vi "File List Window 2.vi"(8 "error in":errorcluster, 9 "File Type":T1=enum."Build Spec (vipb)", 11 "Path":path=path "C:/Users/patrick/AppData/Local/LevyLab/build-support/instruments-vipb--lockin.txt") -> (0 "error out":errorcluster, 1 "File Type out":T1=enum."Build Spec (vipb)", 2 "files out":path[](array[path]), 3 "Path out":path=path "C:/Users/patrick/AppData/Local/LevyLab/build-support/instruments-vipb--lockin.txt")   [LabVIEW 2019, in "Build.lvlib"]
uses:
  Typedefs/Build Type--enum.ctl
  <vilib>/Utility/sysdir.llb/System Directory Type.ctl
  <vilib>/Utility/file.llb/Write Delimited Spreadsheet (string).vi
  <vilib>/Utility/file.llb/Read Delimited Spreadsheet (string).vi
  Build.lvlib
panel:
  in  "Cancel":bool
  in  "OK":bool
  in  "Paths":path[](array[path])
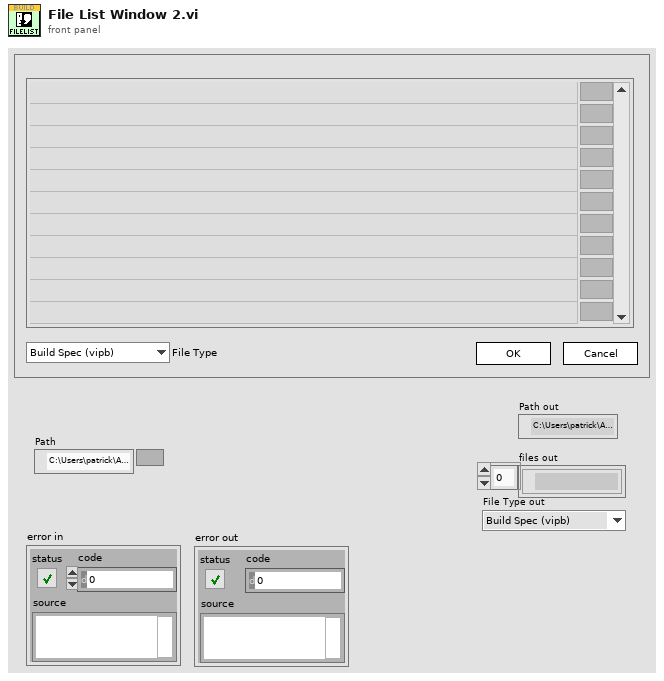
[diagram p1: front panel]
types:
  T1 = typedef "Build.lvlib/Build Type--enum.ctl" = enum16{"LV Project (lvproj)", "Build Spec (vipb)", "Package (vip)"}
  T2 = enum32{"Invalid", "Standard", "Closed", "Hidden", "Minimized", "Maximized"}
  T3 = enum32{"invalid app kind", "Development System", "Run Time System", "Student Edition", "Embedded LabVIEW", "Evaluation", "Custom"}
  T4 = cluster{"Core":cluster{"Current VI Reference":refnum<vi>, "Close Panel on Exit?":bool}, "Path":path, "files":path[], "File Type":T1}
  T5 = typedef "System Directory Type.ctl" = i32
  T6 = cluster{"Current VI Reference":refnum<vi>, "Close Panel on Exit?":bool}
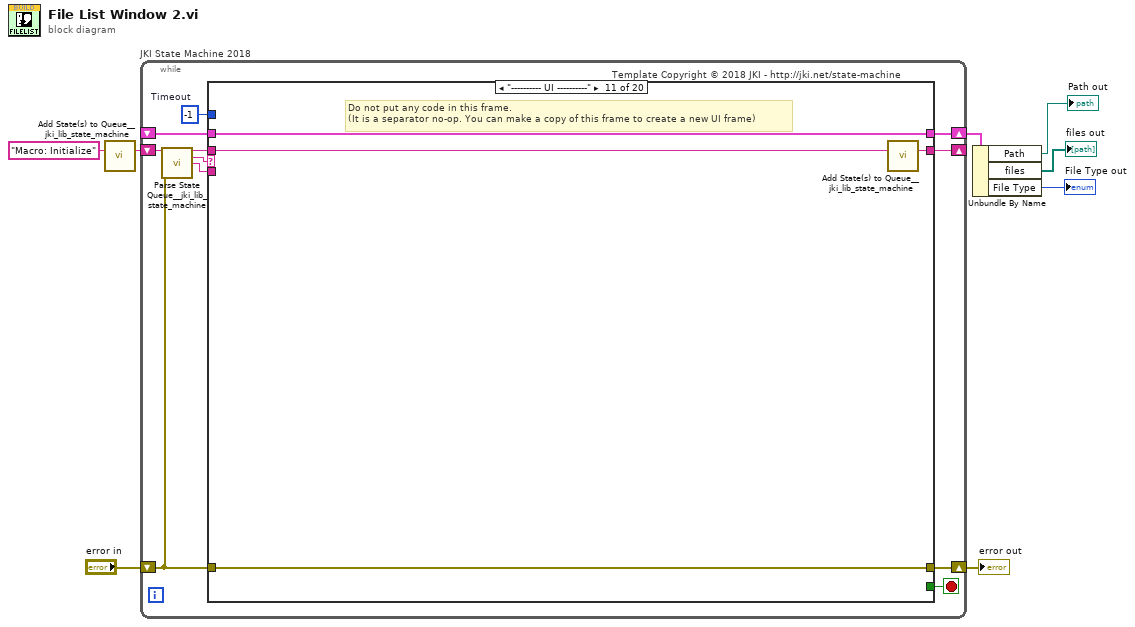
[diagram p0: block diagram]
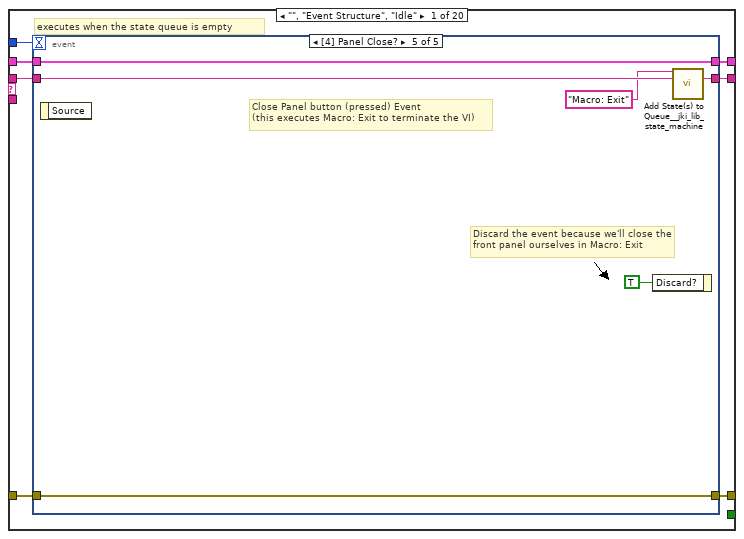
[diagram p2: hidden frame]
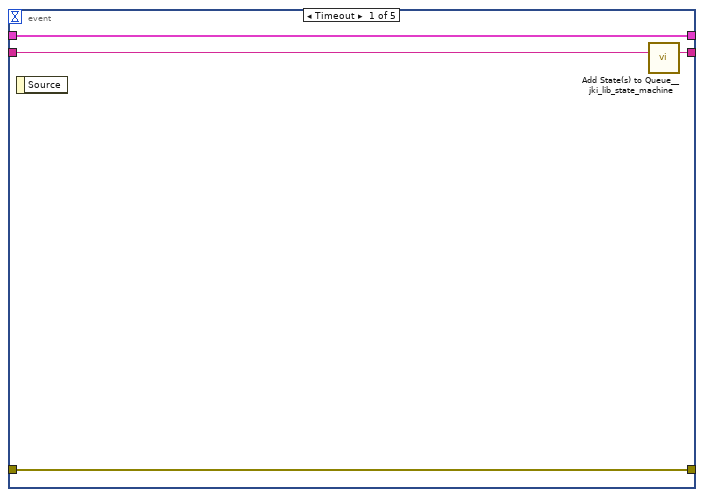
[diagram p3: hidden frame]
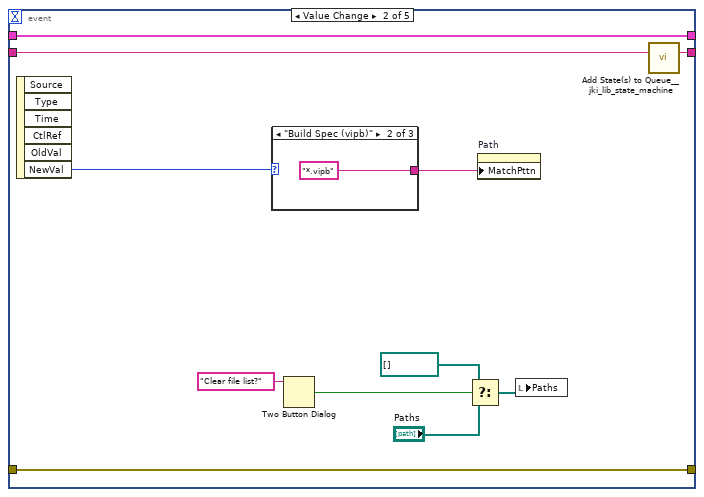
[diagram p4: hidden frame]
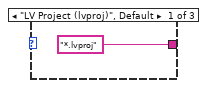
[diagram p5: hidden frame]
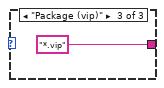
[diagram p6: hidden frame]
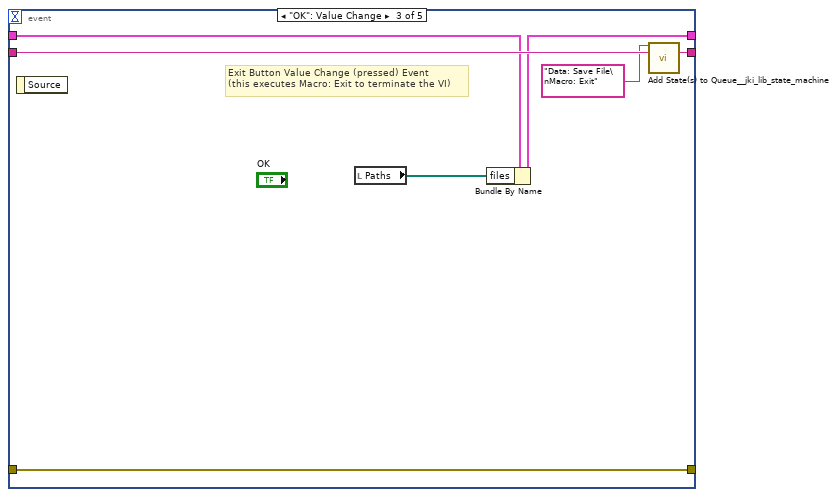
[diagram p7: hidden frame]
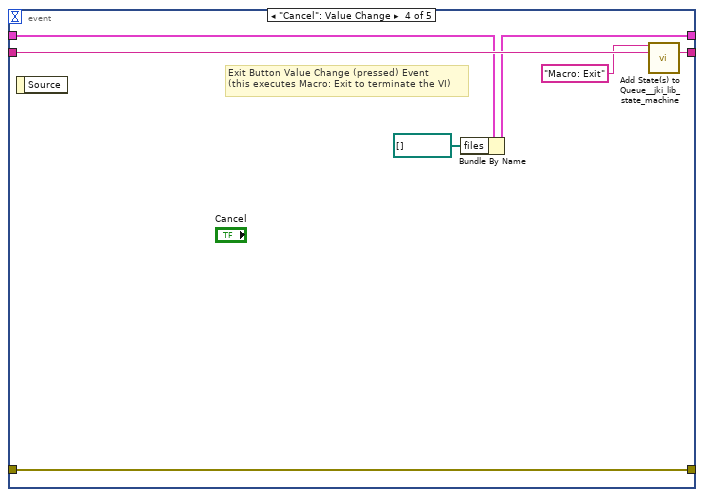
[diagram p8: hidden frame]
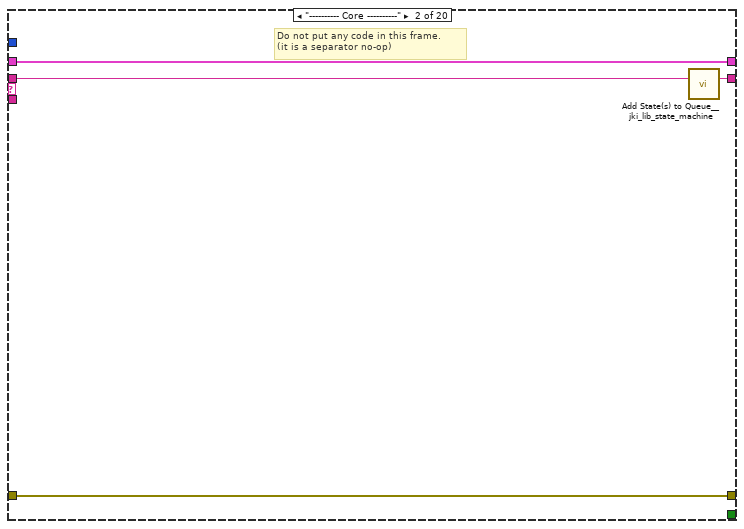
[diagram p9: hidden frame]
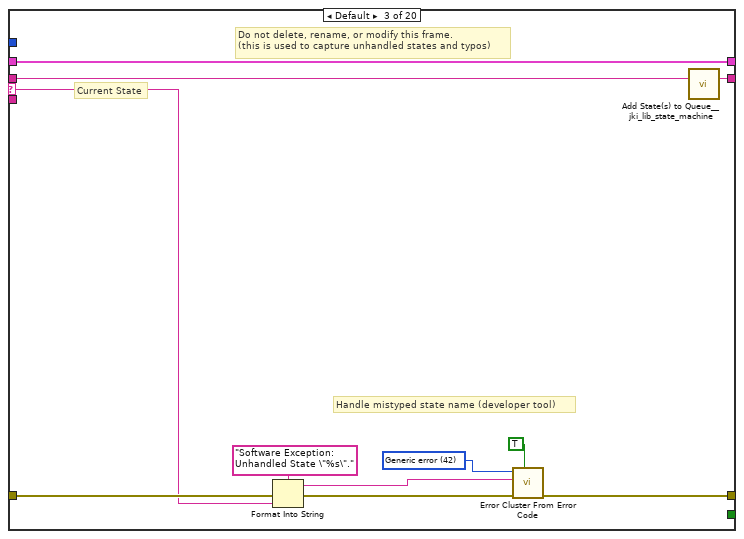
[diagram p10: hidden frame]
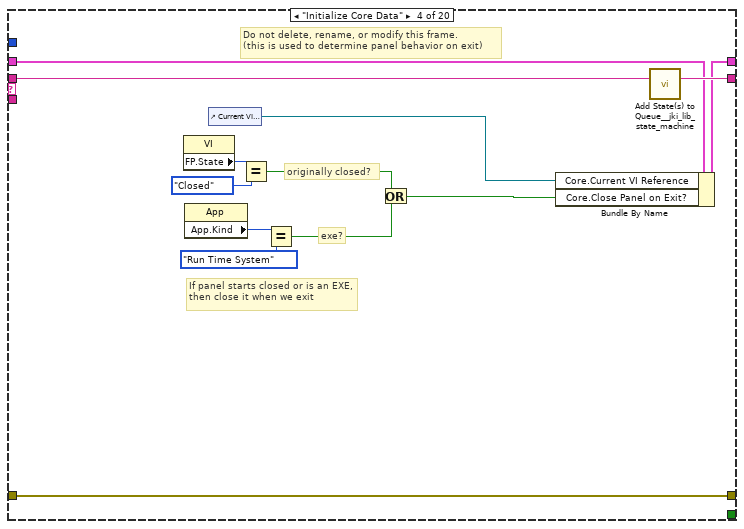
[diagram p11: hidden frame]
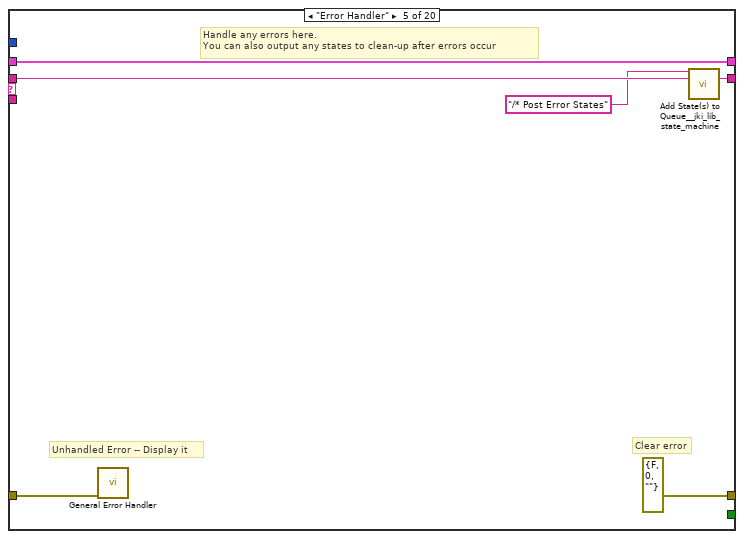
[diagram p12: hidden frame]
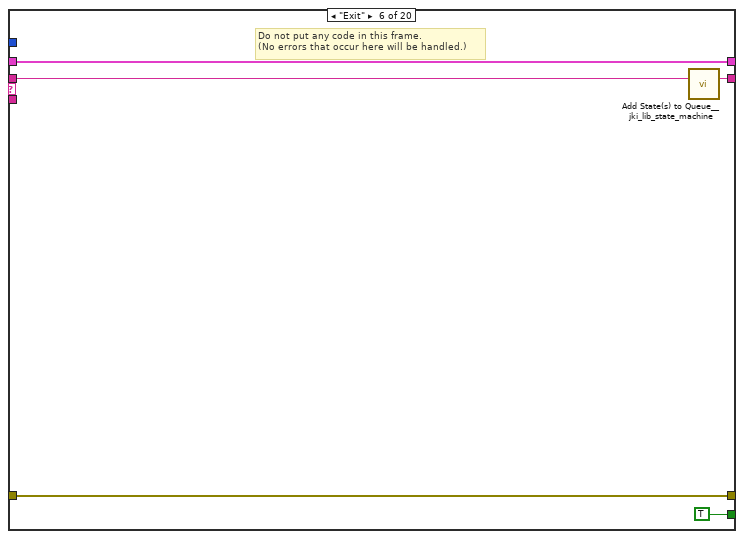
[diagram p13: hidden frame]
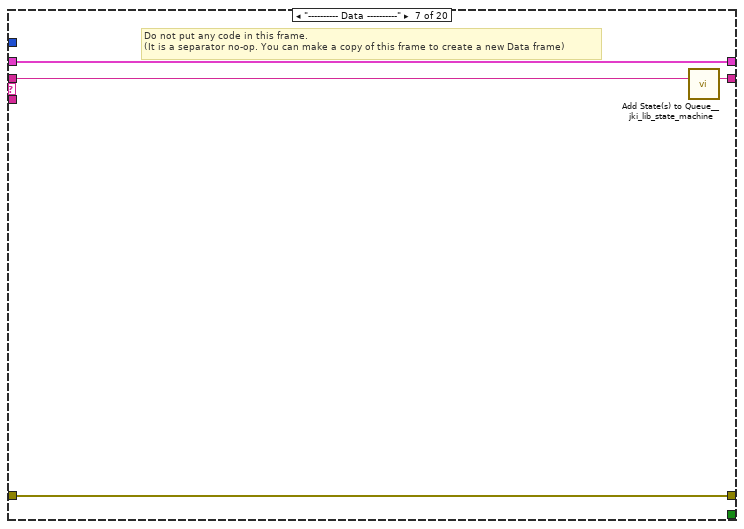
[diagram p14: hidden frame]
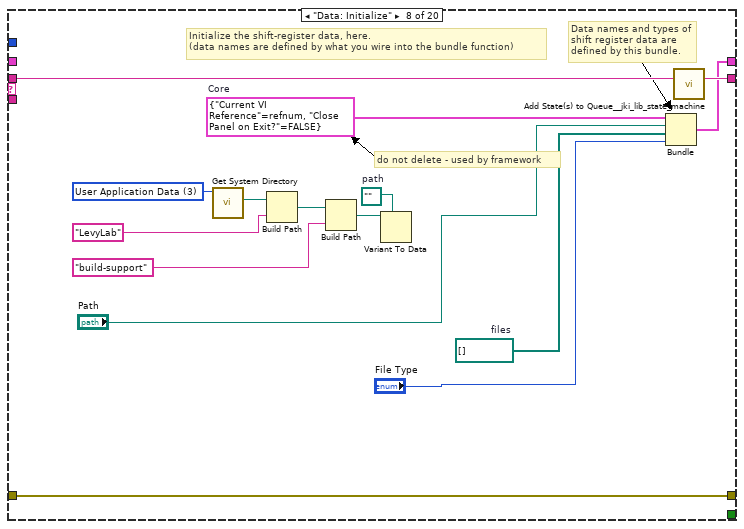
[diagram p15: hidden frame]
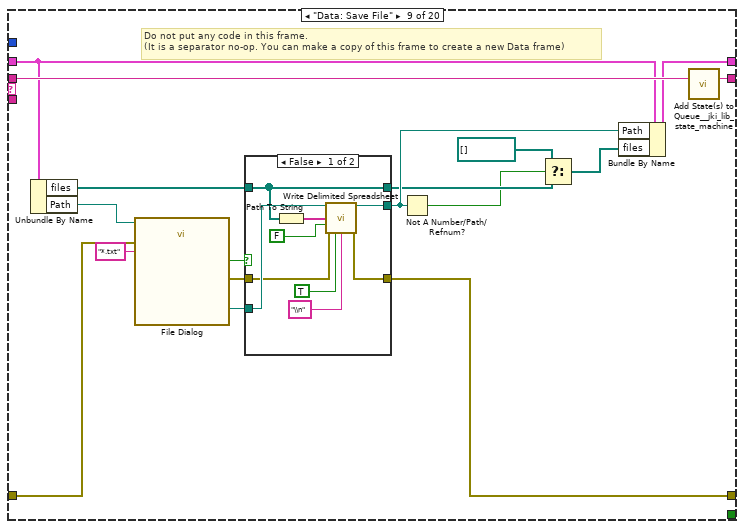
[diagram p16: hidden frame]
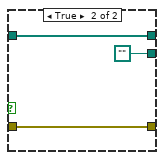
[diagram p17: hidden frame]
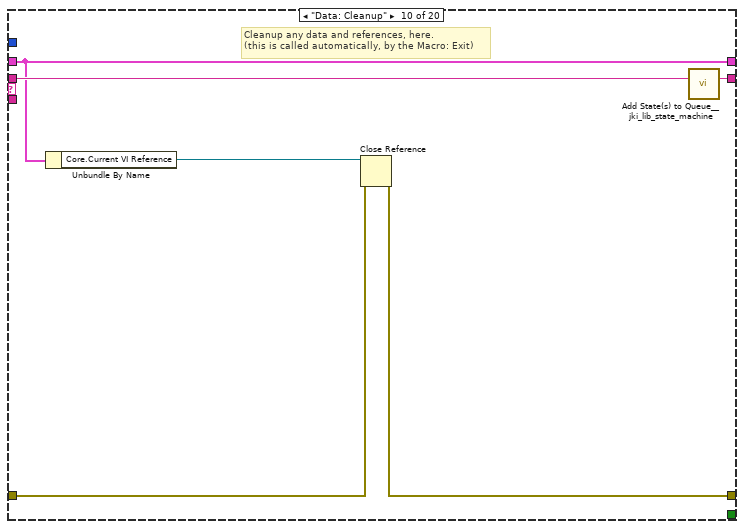
[diagram p18: hidden frame]
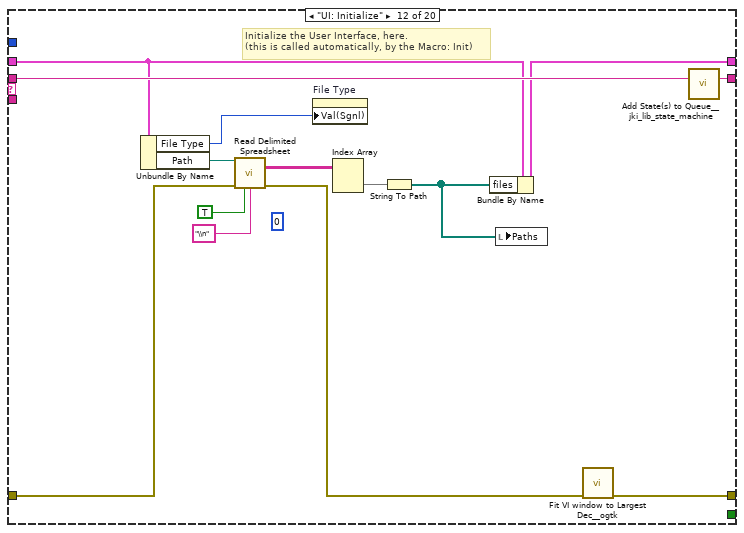
[diagram p19: hidden frame]
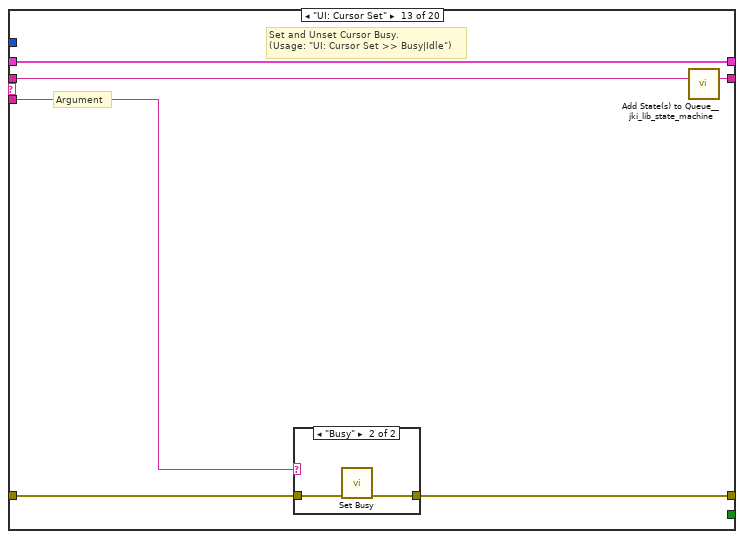
[diagram p20: hidden frame]
diagram:
  n1 = call <vilib>:"Add State(s) to Queue__jki_lib_state_machine.vi"("State(s) in (\"\")"="Macro: Initialize") -> ("States Out"=w8:string)  [unwired: 14 in]
  n2 = while "JKI State Machine 2018" {
    shift-right: [w12] -> w6
    shift-left: _ -> [w11]
    shift-right: [w15] -> w4
    shift-left: "error in" -> [w9]
    shift-right: [w14] -> _
    shift-left: w8 -> [w16]
    stop <- w13 stop-if-true
    w10 = -1  # Timeout
    # "Template Copyright © 2018 JKI - http://jki.net/state-machine"
    n3 = call <vilib>:"Parse State Queue__jki_lib_state_machine.vi"("State Queue"=w16, "Error In (no error)"=w9) -> ("Remaining States"=w18:string, "Current State"=w19:string, "Arguments"=w17:string)  [unwired: 11 in]
    n4 = case shown="\"---------- UI ----------\"" w19 {
      selector: w19 -> [_ _ w69 _ _ _ _ _ _ _ _ _ _ _ _ _ _ _ _ _]
      tunnel: w18 -> [w26 w68 w73 w92 w98 w103 w107 w122 w139 w157 w161 w175 w181 w192 w261 w266 w276 w280 w284 w288]
      tunnel: w17 -> [_ _ _ _ _ _ _ _ _ _ _ _ w176 w186 _ _ _ _ _ _]
      tunnel: w11 -> [w24 w65 w71 w85 w95 w101 w104 _ w135 w152 w158 w164 w179 w188 w258 w263 w273 w277 w281 w285]
      tunnel: [w23 w66 w75 w89 errorcluster {"status"=FALSE, "code"=0, "source"=""} ("error out") w100 w105 w119 w137 w153 w159 w173 w177 w189 w259 w264 w274 w278 w282 w286] -> w15
      tunnel: w9 -> [w22 w66 w74 w89 w94 w100 w105 w119 w127 w154 w159 w167 w178 w190 w259 w264 w274 w278 w282 w286]
      tunnel: [w25 w67 w72 w91 w97 w102 w106 w121 w138 w156 w160 w174 w180 w191 w260 w265 w275 w279 w283 w287] -> w14
      tunnel: [_ _ _ _ _ TRUE _ _ _ _ _ _ _ _ _ _ _ _ _ _] -> w13
      tunnel: [w21 w65 w71 w90 w95 w101 w104 w120 w136 w152 w158 w165 w179 w188 w258 w263 w273 w277 w281 w285] -> w12
      tunnel: w10 -> [w20 _ _ _ _ _ _ _ _ _ _ _ _ _ _ _ _ _ _ _]
      frame "", "Event Structure", "Idle" {
        # "executes when the state queue is empty"
        n5 = event shown="[4] Panel Close?" {
          selector: _ -> [_ _ _ _ _]
          dyn-events: _ -> [_ _ _ _ _]
          timeout: w20 -> [_ _ _ _ _]
          tunnel: w26 -> [w30 w33 w51 w58 w64]
          tunnel: [w29 w41 w50 w57 w63] -> w25
          tunnel: w24 -> [w27 w32 w49 w53 w61]
          tunnel: [w28 w40 w45 w56 w62] -> w23
          tunnel: w22 -> [w28 w40 w45 w56 w62]
          tunnel: [w27 w32 w48 w54 w61] -> w21
          event Timeout {
            n6 = event-data() -> ()  [unwired: 1 in, 1 out]
            n7 = call <vilib>:"Add State(s) to Queue__jki_lib_state_machine.vi"("State(s) in (\"\")"=w30) -> ("States Out"=w29:string)  [unwired: 14 in]
          }
          event Value Change {
            n8 = event-data() -> ("NewVal"=w31:T1)  [unwired: 1 in, 5 out]
            n9 = case shown="\"Build Spec (vipb)\"" w31 {
              tunnel: ["*.lvproj" "*.vipb" "*.vip"] -> w39
              frame "LV Project (lvproj)", Default {
              }
              frame "Build Spec (vipb)" {
              }
              frame "Package (vip)" {
              }
            }
            n10 = Two Button Dialog(message="Clear file list?") -> (T button?=w37:bool)  [unwired: 2 in]
            n11 = Select(t=path[] [] ("f"), s=w37, f="Paths") -> (s? t:f=w36:path[])
            n12 = property on="Path" class="Path"("MatchPttn"=w39) -> ()  [unwired: 2 in, 2 out]
            n13 = local write "Paths"(w36) -> ()
            n14 = call <vilib>:"Add State(s) to Queue__jki_lib_state_machine.vi"("State(s) in (\"\")"=w33) -> ("States Out"=w41:string)  [unwired: 14 in]
          }
          event "OK": Value Change {
            # "Exit Button Value Change (pressed) Event\n(this executes Macro: Exit to terminate the VI)"
            n15 = event-data() -> ()  [unwired: 1 in, 1 out]
            n16 = local read "Paths"() -> (w47:path[])
            n17 = Bundle By Name(cluster=w49, "files"=w47) -> (w48:T4)
            n18 = call <vilib>:"Add State(s) to Queue__jki_lib_state_machine.vi"("State(s) in Front (\"\")"="Data: Save File\nMacro: Exit", "State(s) in (\"\")"=w51) -> ("States Out"=w50:string)  [unwired: 13 in]
          }
          event "Cancel": Value Change {
            # "Exit Button Value Change (pressed) Event\n(this executes Macro: Exit to terminate the VI)"
            n19 = event-data() -> ()  [unwired: 1 in, 1 out]
            n20 = Bundle By Name(cluster=w53, "files"=path[] []) -> (w54:T4)
            n21 = call <vilib>:"Add State(s) to Queue__jki_lib_state_machine.vi"("State(s) in Front (\"\")"="Macro: Exit", "State(s) in (\"\")"=w58) -> ("States Out"=w57:string)  [unwired: 13 in]
          }
          event Panel Close? {
            # "Discard the event because we'll close the front panel ourselves in Macro: Exit"
            # "Close Panel button (pressed) Event\n(this executes Macro: Exit to terminate the VI)"
            n22 = event-data() -> ()  [unwired: 1 in, 1 out]
            n23 = event-data("Discard?"=TRUE) -> ()  [unwired: 1 in, 1 out]
            n24 = call <vilib>:"Add State(s) to Queue__jki_lib_state_machine.vi"("State(s) in Front (\"\")"="Macro: Exit", "State(s) in (\"\")"=w64) -> ("States Out"=w63:string)  [unwired: 13 in]
          }
        }
      }
      frame "---------- Core ----------" {
        # "Do not put any code in this frame.\n(it is a separator no-op)"
        n25 = call <vilib>:"Add State(s) to Queue__jki_lib_state_machine.vi"("State(s) in (\"\")"=w68) -> ("States Out"=w67:string)  [unwired: 14 in]
      }
      frame Default {
        w78 = 42 items=["No error", "Argument error", "Memory is full", "Out of zone", "End of file", "File already open", "Generic file I/O error", "File not found", "File permission error", "Disk is full", "Duplicate path", "Too many files open", "System feature not enabled", "Resource file not found", "Cannot add resource", "Resource not found", "Image not found", "Image memory error", "Pen does not exist", "Config type invalid", "Config token not found", "Config parse error", "Config memory error", "Bad external code format", "Bad external code offset", "External code not present", "Null window", "Destroy window error", "Null menu", "Print aborted", "Bad print record", "Print driver error", "Windows error during printing", "Memory error during printing", "Print dialog error", "Generic print error", "Invalid device refnum", "Device not found", "Device parameter error", "Device unit error", "Cannot open device", "Device call aborted", "Generic error", "Cancelled by user", "Object ID too low", "Object ID too high", "Object not in heap", "Unknown heap", "Unknown object (invalid DefProc)", "Unknown object (DefProc not in table)", "Message out of range", "Invalid (null) method", "Unknown message", "Manager call not supported", "Bad address", "Network operation in progress", "Network operation timed out", "Connection is busy", "Network attribute not supported", "Network error", "Address in use", "System out of memory", "Connection aborted", "Connection refused", "Not connected", "Already connected", "Connection closed", "Initialization error (interapplication manager)", "Bad occurrence", "Wait on unbound occurrence handler", "Occurrence queue overflow", "Datalog type conflict", "Unused", "Unrecognized type (interapplication manager)", "Memory corrupt", "Failed to make temporary DLL", "Old CIN version", "Drag socket not found", "Failed to load drop-object", "Failed to register OLE object", "Failed to release OLE object", "Format specifier type mismatch", "Unknown format specifier", "Too few format specifiers", "Too many format specifiers", "Scan failed", "Newer CIN version", "Error converting to variant", "Runtime menu error", "Password tampered", "Variant attribute not found", "Incompatible variant data type", "Event data is not available", "Event Store is not present", "Occurrence is not found", "Event Queue is not created", "Event info is not available", "Refnum passed is NULL", "Error retrieving Class GUID", "Error retrieving CoClass GUID", "Error retrieving TypeLib GUID.", "Bad built application magic bytes.", "Specific driver is different from the specific driver associated with the Logical Name.", "There is no session opened to the class driver.", "Max Error", "MAX - Error with config objects", "MAX - Error loading configuration", "MAX - Group not supported"]
        # "Current State"
        # "Do not delete, rename, or modify this frame.\n(this is used to capture unhandled states and typos)"
        # "Handle mistyped state name (developer tool)"
        n26 = Format Into String(format string="Software Exception: Unhandled State \"%s\"." ("message"), error in=w74, w69) -> (resulting string=w77:string, error out=w76:errorcluster)  [unwired: 1 in]
        n27 = call <vilib>:"Error Cluster From Error Code.vi"("show call chain? (False)"=TRUE, "error in (no error)"=w76, "error message (\"\")"=w77, "error code (0)"=w78) -> ("error out"=w75:errorcluster)  [unwired: 5 in]
        n28 = call <vilib>:"Add State(s) to Queue__jki_lib_state_machine.vi"("State(s) in (\"\")"=w73) -> ("States Out"=w72:string)  [unwired: 14 in]
      }
      frame "Initialize Core Data" {
        # "Do not delete, rename, or modify this frame.\n(this is used to determine panel behavior on exit)"
        # "originally closed?"
        # "exe?"
        # "If panel starts closed or is an EXE, then close it when we exit"
        n29 = property class="VI"() -> ("FP.State"=w82:T2)  [unwired: 2 in, 2 out]
        n30 = property class="App"() -> ("App.Kind"=w88:T3)  [unwired: 2 in, 2 out]
        n31 = control-ref of="Current VI Reference"() -> (w83:refnum<vi>)
        n32 = Equal?(x=w82, y=T2."Closed" ("Front Panel Window:State")) -> (x = y?=w80:bool)
        n33 = Equal?(x=w88, y=T3."Run Time System" ("Application:Kind")) -> (x = y?=w86:bool)
        n34 = Or(x=w80, y=w86) -> (x .or. y?=w84:bool)
        n35 = Bundle By Name(cluster=w85, "Core.Current VI Reference"=w83, "Core.Close Panel on Exit?"=w84) -> (w90:T4)
        n36 = call <vilib>:"Add State(s) to Queue__jki_lib_state_machine.vi"("State(s) in (\"\")"=w92) -> ("States Out"=w91:string)  [unwired: 14 in]
      }
      frame "Error Handler" {
        # "Unhandled Error -- Display it"
        # "Handle any errors here.\nYou can also output any states to clean-up after errors occur"
        # "Clear error"
        n37 = call <vilib>:"General Error Handler.vi"("error in (no error)"=w94) -> ()  [unwired: 10 in, 5 out]
        n38 = call <vilib>:"Add State(s) to Queue__jki_lib_state_machine.vi"("State(s) in Front (\"\")"="/* Post Error States", "State(s) in (\"\")"=w98) -> ("States Out"=w97:string)  [unwired: 13 in]
      }
      frame "Exit" {
        # "Do not put any code in this frame.\n(No errors that occur here will be handled.)"
        n39 = call <vilib>:"Add State(s) to Queue__jki_lib_state_machine.vi"("State(s) in (\"\")"=w103) -> ("States Out"=w102:string)  [unwired: 14 in]
      }
      frame "---------- Data ----------" {
        # "Do not put any code in this frame.\n(It is a separator no-op. You can make a copy of this frame to create a new Data frame)"
        n40 = call <vilib>:"Add State(s) to Queue__jki_lib_state_machine.vi"("State(s) in (\"\")"=w107) -> ("States Out"=w106:string)  [unwired: 14 in]
      }
      frame "Data: Initialize" {
        w110 = path ""  # path
        w116 = T5 3 items=["User Home"=0, "User Desktop"=1, "User Documents"=2, "User Application Data"=3, "User Preferences"=4, "User Temporary"=5, "Public Documents"=6, "Public Application Data"=7, "Public Preferences"=8, "Public Cache"=13, "System Core Libraries"=9, "System Installed Libraries"=10, "Application Files"=11, "Boot Volume Root"=12] ("system directory type")
        w117 = path[] []  # files
        w118 = T6 {"Current VI Reference"=refnum, "Close Panel on Exit?"=FALSE}  # Core
        # "do not delete - used by framework"
        # "Data names and types of shift register data are defined by this bundle."
        # "Initialize the shift-register data, here.\n(data names are defined by what you wire into the bundle function)"
        n41 = call <vilib>:"Get System Directory.vi"("system directory type"=w116) -> ("system directory"=w114:path)  [unwired: 10 in]
        n42 = Build Path(base path=w114, name or relative path="LevyLab") -> (appended path=w113:path)
        n43 = Build Path(base path=w113, name or relative path="build-support") -> (appended path=w111:path)
        n44 = Variant To Data(type=w110, Variant=w111) -> ()  [unwired: 1 in, 2 out]
        n45 = Bundle("Core"=w118, "Path"="Path", "files"=w117, "File Type"="File Type") -> (w120:T4)  [unwired: 1 in]
        n46 = call <vilib>:"Add State(s) to Queue__jki_lib_state_machine.vi"("State(s) in (\"\")"=w122) -> ("States Out"=w121:string)  [unwired: 14 in]
      }
      frame "Data: Save File" {
        # "Do not put any code in this frame.\n(It is a separator no-op. You can make a copy of this frame to create a new Data frame)"
        n47 = Unbundle By Name(w135) -> ("files"=w125:path[], "Path"=w130:path)
        n48 = call "File Dialog"("start path"=w130, "error in"=w127, "pattern (all files)"="*.txt") -> ("selected path"=w129:path, "cancelled"=w126:bool, "error out"=w128:errorcluster)  [unwired: 9 in, 1 out]
        n49 = case shown="False" w126 {
          tunnel: [w141 w151] -> w137
          tunnel: [w145 path ""] -> w132
          tunnel: w129 -> [w143 _]
          tunnel: w128 -> [w140 w151]
          tunnel: w125 -> [w142 w149]
          tunnel: [w142 w149] -> w124
          frame False {
            n50 = Path To String(path=w142) -> (string=w148:string[])
            n51 = call-poly <vilib>:"Write Delimited Spreadsheet.vi"("file path (dialog if empty)"=w143, "1D data"=w148, "append to file? (new file:F)"=FALSE, "error in (no error)"=w140, "transpose? (no:F)"=TRUE, "delimiter (\\t)"="\\n" ("delimiter (\\t)")) -> ("new file path (Not A Path if cancelled)"=w145:path, "error out"=w141:errorcluster)  [unwired: 8 in]
          }
          frame True {
          }
        }
        n52 = Not A Number/Path/Refnum?(number/path/refnum=w132) -> (NaN/Path/Refnum?=w123:bool)
        n53 = Select(t=path[] [] ("files"), s=w123, f=w124) -> (s? t:f=w133:path[])
        n54 = Bundle By Name(cluster=w135, "Path"=w132, "files"=w133) -> (w136:T4)
        n55 = call <vilib>:"Add State(s) to Queue__jki_lib_state_machine.vi"("State(s) in (\"\")"=w139) -> ("States Out"=w138:string)  [unwired: 14 in]
      }
      frame "Data: Cleanup" {
        # "Cleanup any data and references, here.\n(this is called automatically, by the Macro: Exit)"
        n56 = Unbundle By Name(w152) -> ("Core.Current VI Reference"=w155:refnum<vi>)
        n57 = Close Reference(reference=w155, error in (no error)=w154) -> (error out=w153:errorcluster)
        n58 = call <vilib>:"Add State(s) to Queue__jki_lib_state_machine.vi"("State(s) in (\"\")"=w157) -> ("States Out"=w156:string)  [unwired: 14 in]
      }
      frame "---------- UI ----------" {
        # "Do not put any code in this frame.\n(It is a separator no-op. You can make a copy of this frame to create a new UI frame)"
        n59 = call <vilib>:"Add State(s) to Queue__jki_lib_state_machine.vi"("State(s) in (\"\")"=w161) -> ("States Out"=w160:string)  [unwired: 14 in]
      }
      frame "UI: Initialize" {
        (unwired) 0 ("disabled index (col)")
        # "Initialize the User Interface, here.\n(this is called automatically, by the Macro: Init)"
        n60 = Unbundle By Name(w164) -> ("File Type"=w162:T1, "Path"=w169:path)
        n61 = call-poly <vilib>:"Read Delimited Spreadsheet.vi"("file path (dialog if empty)"=w169, "error in (no error)"=w167, "transpose? (F)"=TRUE, "delimiter (\\t)"="\\n" ("delimiter (\\t)")) -> ("all rows"=w168:string[][], "error out"=w166:errorcluster)  [unwired: 6 in, 4 out]
        n62 = property on="File Type" class="Enum (strict)"("Val(Sgnl)"=w162) -> ()  [unwired: 2 in, 2 out]
        n63 = Index Array(array=w168) -> (element=w171:string[])  [unwired: 2 in]
        n64 = String To Path(string=w171) -> (path=w163:path[])
        n65 = Bundle By Name(cluster=w164, "files"=w163) -> (w165:T4)
        n66 = local write "Paths"(w163) -> ()
        n67 = call <userlib>:"Fit VI window to Largest Dec__ogtk.vi"("error in (no error)"=w166) -> ("error out"=w173:errorcluster)  [unwired: 5 in, 1 out]
        n68 = call <vilib>:"Add State(s) to Queue__jki_lib_state_machine.vi"("State(s) in (\"\")"=w175) -> ("States Out"=w174:string)  [unwired: 14 in]
      }
      frame "UI: Cursor Set" {
        # "Argument"
        # "Set and Unset Cursor Busy.\n(Usage: \"UI: Cursor Set >> Busy|Idle\")"
        n69 = case shown="\"Busy\"" w176 {
          tunnel: w178 -> [w183 w185]
          tunnel: [w182 w184] -> w177
          frame "Idle", Default {
            n70 = call <vilib>:"Unset Busy.vi"("error in (no error)"=w183) -> ("error out"=w182:errorcluster)  [unwired: 10 in]
          }
          frame "Busy" {
            n71 = call <vilib>:"Set Busy.vi"("error in (no error)"=w185) -> ("error out"=w184:errorcluster)  [unwired: 9 in, 1 out]
          }
        }
        n72 = call <vilib>:"Add State(s) to Queue__jki_lib_state_machine.vi"("State(s) in (\"\")"=w181) -> ("States Out"=w180:string)  [unwired: 14 in]
      }
      frame "UI: Front Panel State" {
        # "Argument"
        # "Set Front Panel Open or Closed\n(Usage: \"UI: Front Panel State >> Open|Close\")"
        n73 = Unbundle By Name(w188) -> ("Core.Current VI Reference"=w187:refnum<vi>)
        n74 = case shown="\"Minimize\", \"Minimized\"" w186 {
          tunnel: w190 -> [w198 w213 w224 w237 w250]
          tunnel: [w200 w214 w226 w239 w252] -> w189
          tunnel: w187 -> [w199 w211 w225 w238 w251]
          frame "Open", "Standard", Default {
            w193 = T2."Standard" ("State")
            n75 = property class="VI"(reference=w199, error in=w198) -> (reference out=w196:refnum<vi>, error out=w197:errorcluster, "FP.State"=w195:T2)
            n76 = Not Equal?(x=w195, y=w193) -> (x != y?=w194:bool)
            n77 = case shown="True" w194 {
              tunnel: [w204 w206] -> w200
              tunnel: w197 -> [w203 w206]
              tunnel: w196 -> [w202 _]
              tunnel: w193 -> [w201 _]
              frame True {
                n78 = invoke class="VI" method="FP.Open"(reference=w202, error in=w203, "Activate"=TRUE, "State"=w201) -> (error out=w204:errorcluster)  [unwired: 1 in, 4 out]
              }
              frame False {
              }
            }
          }
          frame "Close", "Closed" {
            n79 = property class="VI"(reference=w211, error in=w213) -> (reference out=w210:refnum<vi>, error out=w212:errorcluster, "FP.State"=w208:T2)
            n80 = Not Equal?(x=w208, y=T2."Closed" ("Front Panel Window:State")) -> (x != y?=w207:bool)
            n81 = case shown="True" w207 {
              tunnel: [w215 w218] -> w214
              tunnel: w212 -> [w215 w217]
              tunnel: w210 -> [_ w216]
              frame False {
              }
              frame True {
                n82 = invoke class="VI" method="FP.Close"(reference=w216, error in=w217) -> (error out=w218:errorcluster)  [unwired: 1 in, 2 out]
              }
            }
          }
          frame "Hidden", "Hide" {
            w219 = T2."Hidden" ("State")
            n83 = property class="VI"(reference=w225, error in=w224) -> (reference out=w222:refnum<vi>, error out=w223:errorcluster, "FP.State"=w221:T2)
            n84 = Not Equal?(x=w221, y=w219) -> (x != y?=w220:bool)
            n85 = case shown="True" w220 {
              tunnel: [w230 w231] -> w226
              tunnel: w223 -> [w229 w231]
              tunnel: w222 -> [w228 _]
              tunnel: w219 -> [w227 _]
              frame True {
                n86 = invoke class="VI" method="FP.Open"(reference=w228, error in=w229, "State"=w227) -> (error out=w230:errorcluster)  [unwired: 2 in, 4 out]
              }
              frame False {
              }
            }
          }
          frame "Minimize", "Minimized" {
            w232 = T2."Minimized" ("State")
            n87 = property class="VI"(reference=w238, error in=w237) -> (reference out=w235:refnum<vi>, error out=w236:errorcluster, "FP.State"=w234:T2)
            n88 = Not Equal?(x=w234, y=w232) -> (x != y?=w233:bool)
            n89 = case shown="True" w233 {
              tunnel: [w243 w244] -> w239
              tunnel: w236 -> [w242 w244]
              tunnel: w235 -> [w241 _]
              tunnel: w232 -> [w240 _]
              frame True {
                n90 = invoke class="VI" method="FP.Open"(reference=w241, error in=w242, "State"=w240) -> (error out=w243:errorcluster)  [unwired: 2 in, 4 out]
              }
              frame False {
              }
            }
          }
          frame "Maximize", "Maximized" {
            w245 = T2."Maximized" ("State")
            n91 = property class="VI"(reference=w251, error in=w250) -> (reference out=w248:refnum<vi>, error out=w249:errorcluster, "FP.State"=w247:T2)
            n92 = Not Equal?(x=w247, y=w245) -> (x != y?=w246:bool)
            n93 = case shown="True" w246 {
              tunnel: [w256 w257] -> w252
              tunnel: w249 -> [w255 w257]
              tunnel: w248 -> [w254 _]
              tunnel: w245 -> [w253 _]
              frame True {
                n94 = invoke class="VI" method="FP.Open"(reference=w254, error in=w255, "State"=w253) -> (error out=w256:errorcluster)  [unwired: 2 in, 4 out]
              }
              frame False {
              }
            }
          }
        }
        n95 = call <vilib>:"Add State(s) to Queue__jki_lib_state_machine.vi"("State(s) in (\"\")"=w192) -> ("States Out"=w191:string)  [unwired: 14 in]
      }
      frame "---------- Macro ----------" {
        # "Do not put any code in this frame.\n(It is a separator no-op. You can make a copy of this frame to create a new Macro frame)"
        n96 = call <vilib>:"Add State(s) to Queue__jki_lib_state_machine.vi"("State(s) in (\"\")"=w261) -> ("States Out"=w260:string)  [unwired: 14 in]
      }
      frame "Macro: Initialize" {
        w262 = "Data: Initialize\nInitialize Core Data\nUI: Initialize\nUI: Front Panel State >> Open"  # Data: Initialize Initialize Core Data UI: Initialize UI: Front Panel State >> Open
        # "Initialization Macro\n(This is called once, when the VI starts)"
        n97 = call <vilib>:"Add State(s) to Queue__jki_lib_state_machine.vi"("State(s) in Front (\"\")"=w262, "State(s) in (\"\")"=w266) -> ("States Out"=w265:string)  [unwired: 13 in]
      }
      frame "Macro: Exit" {
        # "Exit Macro\n(This is called once, when the VI exits)"
        n98 = Unbundle By Name(w273) -> ("Core.Close Panel on Exit?"=w272:bool)
        n99 = Select(t="UI: Front Panel State >> Close", s=w272, f="") -> (s? t:f=w269:string)
        n100 = call <vilib>:"Add State(s) to Queue__jki_lib_state_machine.vi"("State(s) in (\"\")"=w269, "State(s) at Back (\"\")"="Data: Cleanup\nExit") -> ("States Out"=w267:string)  [unwired: 13 in]
        n101 = call <vilib>:"Add State(s) to Queue__jki_lib_state_machine.vi"("State(s) in Front (\"\")"=w267, "State(s) in (\"\")"=w276) -> ("States Out"=w275:string)  [unwired: 13 in]
      }
      frame "---------- New Category ----------" {
        # "Template Separator\n(You can make a copy of, or modify, this frame)"
        n102 = call <vilib>:"Add State(s) to Queue__jki_lib_state_machine.vi"("State(s) in (\"\")"=w280) -> ("States Out"=w279:string)  [unwired: 14 in]
      }
      frame "New Category: 1" {
        # "Your code here.\n(You can make a copy of, or modify, this frame)"
        n103 = call <vilib>:"Add State(s) to Queue__jki_lib_state_machine.vi"("State(s) in (\"\")"=w284) -> ("States Out"=w283:string)  [unwired: 14 in]
      }
      frame "New Category: 2" {
        # "Your code here.\n(You can make a copy of, or modify, this frame)"
        n104 = call <vilib>:"Add State(s) to Queue__jki_lib_state_machine.vi"("State(s) in (\"\")"=w288) -> ("States Out"=w287:string)  [unwired: 14 in]
      }
    }
  }
  "error out" <- w4
  n105 = Unbundle By Name(w6) -> ("Path"=→"Path out":path, "files"=→"files out":path[], "File Type"=→"File Type out":T1)
